vi "Start And Count.vi"(10 "indices":u64[](array[numeric]), 11 "Variant":variant) -> (2 "count":u64[](array[numeric]), 3 "start":u64[](array[numeric]))   [LabVIEW 2019]
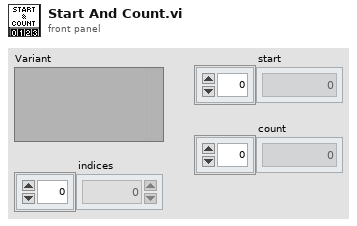
[diagram p1: front panel]
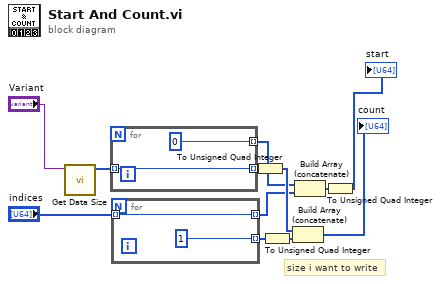
[diagram p0: block diagram]
diagram:
  # "size i want to write"
  n1 = call "Get Data Size.vi"("Variant"="Variant") -> ("size"=w2:u32[])  [unwired: 8 in, 2 out]
  n2 = for {
    tunnel: w2 -> [w13] mode=indexing
    tunnel: [0] -> w5 mode=indexing
    tunnel: [w13] -> w7 mode=indexing
  }
  n3 = for {
    tunnel: "indices" -> [w16] mode=indexing
    tunnel: [w16] -> w4 mode=indexing
    tunnel: [1] -> w6 mode=indexing
  }
  n4 = To Unsigned Quad Integer(1:w7) -> (0:w9:u64[])
  n5 = To Unsigned Quad Integer(1:w6) -> (0:w8:u64[])
  n6 = Build Array (concatenate)(w9, w8) -> (→"count":u64[])
  n7 = Build Array (concatenate)(w5, w4) -> (w11:u64[])
  n8 = To Unsigned Quad Integer(1:w11) -> (0:→"start":u64[])
